vi "Part Type to Weight Type.vi"(8 "error in":errorcluster, 11 "Weight Type":T1) -> (0 "error out":errorcluster, 3 "Part Type":T2)   [LabVIEW 2011]
uses:
  Config Manager Class/Type Definitions/Part Type.ctl
  Config Manager Class/Type Definitions/Weight Type.ctl
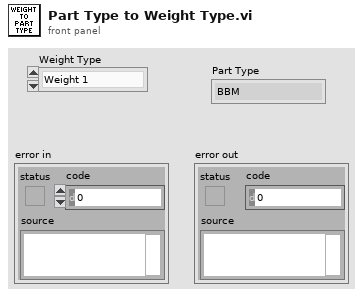
[diagram p1: front panel]
types:
  T1 = typedef "Weight Type.ctl" = enum16{"Weight 1", "Weight 2", "Weight 3", "Weight 4", "Weight 5", "Weight 6", "Weight 7", "Weight 8"}
  T2 = typedef "Part Type.ctl" = enum16{"BBM", "HDI", "BARE HDI", "GLUERESERVOIR", "STAMP_1", "STAMP_2", "STAMP_3", "STAMP_4", "STAMP_5", "WEIGHT_1", "WEIGHT_2", "WEIGHT_3", "WEIGHT_4", "WEIGHT_5", "WEIGHT_6", "WEIGHT_7", "WEIGHT_8", "PICKER_TOOL", "GRABER_TOOL"}
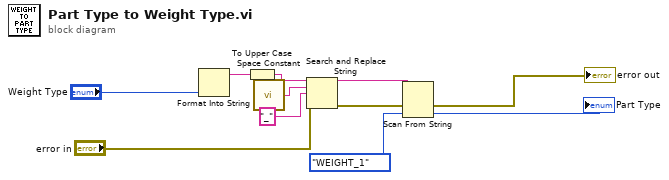
[diagram p0: block diagram]
diagram:
  n1 = Format Into String("Weight Type") -> (resulting string=w9:string)  [unwired: 3 in, 1 out]
  n2 = To Upper Case(1:w9) -> (0:w8:string)
  n3 = call <vilib>:"Space Constant.vi"() -> ("String"=w7:string)
  n4 = Search and Replace String(input string=w8, search string=w7, replace string="_" ("replace string (\"\")"), error in="error in") -> (result string=w2:string, error out=w4:errorcluster)  [unwired: 4 in, 2 out]
  n5 = Scan From String(input string=w2, error in=w4, default 1=Part_Type."WEIGHT_1" ("Part Type")) -> (error out=→"error out":errorcluster, output 1=→"Part Type":T2)  [unwired: 2 in, 2 out]
